vi "SendToSMGRHB.vi"(6 "error in":errorcluster, 7 "meas_point":i32=7, 10 "URL":string="http://smgr.alwaysdata.net/heartbeat/", 11 "date":string="2011-03-24 19:37:00") -> (0 "error out":errorcluster, 2 "body":string="ok", 3 "headers":string="HTTP/1.1 100 Continue\r\n\r\nHTTP/1.1 200 OK\r\nDate: Thu, 24 Mar 2011 13:37:49 GMT\r\nServer: Apache/2.2\r\nVary: Accept-Language,Cookie,User-Agent,Accept-Encoding\r\nContent-Language: en-us\r\nTransfer-Encoding: chunked\r\nContent-Type: text/html; charset=utf-8\r\n\r\n")   [LabVIEW 2010]
uses:
  <vilib>/httpClient/MultipartData.ctl
  <vilib>/httpClient/LabVIEWHTTPClient.lvlib
panel:
  in  "Tab Control":enum32{"Page 1", "Page 2"}(tab)
  out "Array":T1[](array[typedef])=[{"Name"="meas_point", "Value"="7", "File"=path "", "Filename"="", "MIME type"="application/octet-stream"}, {"Name"="date", "Value"="2011-03-24 19:37:00", "File"=path "", "Filename"="", "MIME type"="application/octet-stream"}] caption="Данные для формы"
  # "Измеритель сообщает серверу \nо готовности\n----------------------------------------\nЕсли в ответе, в хедерсе есть \nстрока \"HTTP/1.1 200 OK\"\nзначит всё действительно\nсделано правильно"
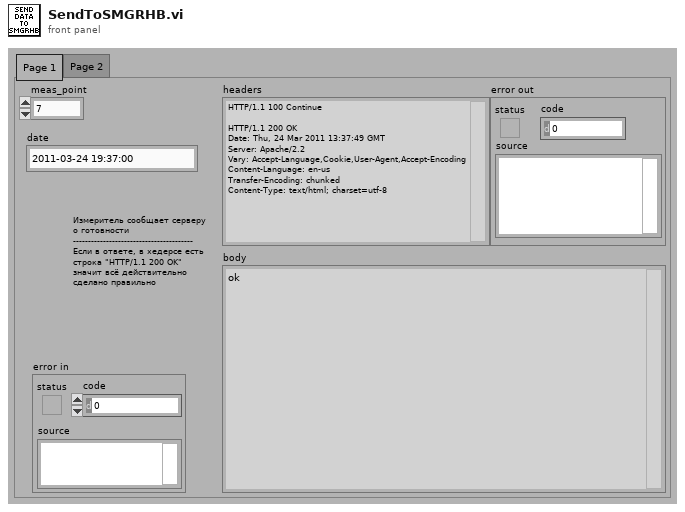
[diagram p1: front panel]
types:
  T1 = typedef "LabVIEWHTTPClient.lvlib/MultipartData.ctl" = cluster{"Name":string, "Value":string, "File":path, "Filename":string, "MIME type":string}
  T2 = typedef "LabVIEWHTTPClient.lvlib/ClientHandle.ctl" = refnum<k1>
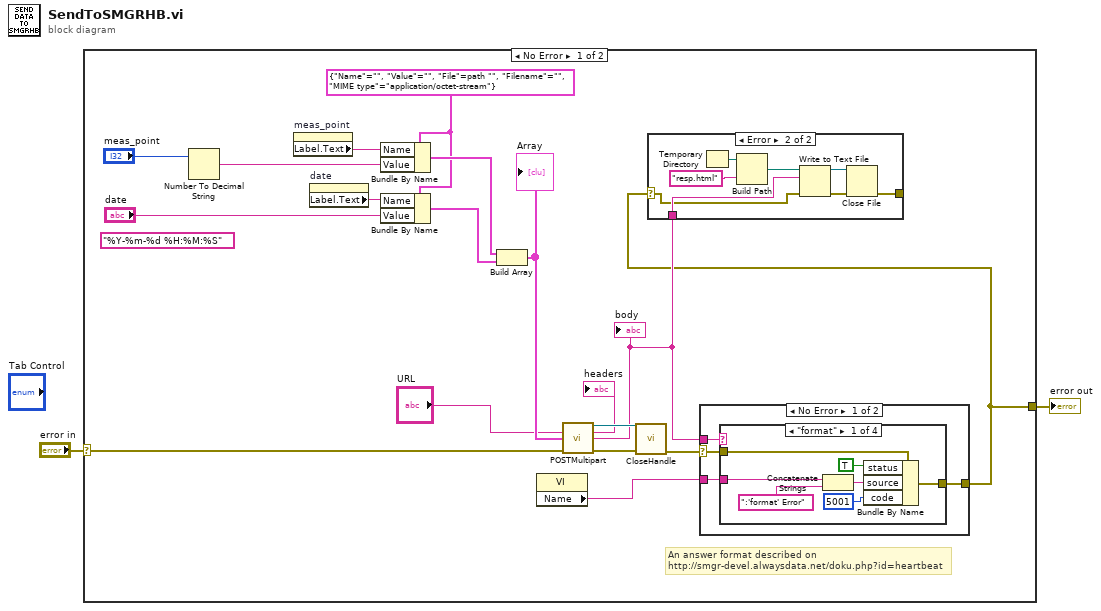
[diagram p0: block diagram]
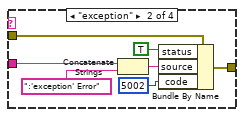
[diagram p2: hidden frame]
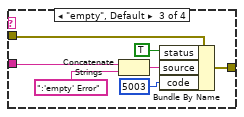
[diagram p3: hidden frame]
diagram:
  n1 = case shown="No Error" "error in" {
    selector: "error in" -> [w13 w57]
    tunnel: [w3 w57] -> w1
    frame No Error {
      w9 = T1 {"Name"="", "Value"="", "File"=path "", "Filename"="", "MIME type"="application/octet-stream"} ("postData")
      (unwired) "%Y-%m-%d %H:%M:%S" ("time format string (%c)")
      # "An answer format described on\nhttp://smgr-devel.alwaysdata.net/doku.php?id=heartbeat"
      n2 = Number To Decimal String(number="meas_point") -> (decimal integer string=w18:string)  [unwired: 1 in]
      n3 = property on="meas_point" class="DigNum (strict)"() -> ("Label.Text"=w15:string)  [unwired: 2 in, 2 out]
      n4 = property on="date" class="Str"() -> ("Label.Text"=w14:string)  [unwired: 2 in, 2 out]
      n5 = Bundle By Name(cluster=w9, "Name"=w15, "Value"=w18) -> (w20:T1)
      n6 = Bundle By Name(cluster=w9, "Name"=w14, "Value"="date") -> (w19:T1)
      n7 = Build Array(w20, w19) -> (w8:T1[])
      "Array" <- w8
      n8 = property on="Property Node" class="VI"() -> ("Name"=w4:string)  [unwired: 2 in, 2 out]
      n9 = call <vilib>:"POSTMultipart.vi"("URL"="URL", "data"=w8, "error in (no error)"=w13) -> ("client handle out"=w12:T2, "headers"=→"headers":string, "body"=w5:string, "error out"=w10:errorcluster)  [unwired: 9 in]
      "body" <- w5
      n10 = call <vilib>:"CloseHandle.vi"("client handle"=w12, "error in (no error)"=w10) -> ("error out"=w6:errorcluster)  [unwired: 13 in]
      n11 = case shown="No Error" w6 {
        selector: w6 -> [w23 w47]
        tunnel: [w22 w47] -> w3
        tunnel: w5 -> [w24 _]
        tunnel: w4 -> [w21 _]
        frame No Error {
          n12 = case shown="\"format\"" w24 {
            tunnel: w23 -> [w29 w33 w41 w46]
            tunnel: [w30 w32 w39 w46] -> w22
            tunnel: w21 -> [w31 w34 w40 _]
            frame "format" {
              n13 = Concatenate Strings(w31, ":'format' Error") -> (w26:string)
              n14 = Bundle By Name(cluster=w29, "status"=TRUE, "source"=w26, "code"=5001) -> (w30:errorcluster)
            }
            frame "exception" {
              n15 = Concatenate Strings(w34, ":'exception' Error") -> (w37:string)
              n16 = Bundle By Name(cluster=w33, "status"=TRUE, "source"=w37, "code"=5002) -> (w32:errorcluster)
            }
            frame "empty", Default {
              n17 = Concatenate Strings(w40, ":'empty' Error") -> (w44:string)
              n18 = Bundle By Name(cluster=w41, "status"=TRUE, "source"=w44, "code"=5003) -> (w39:errorcluster)
            }
            frame "ok" {
            }
          }
        }
        frame Error {
        }
      }
      n19 = case shown="Error" w3 {
        selector: w3 -> [w48 w49]
        tunnel: w5 -> [_ w51]
        tunnel: [w48 w50] -> _
        frame No Error {
        }
        frame Error {
          n20 = Temporary Directory() -> (w56:path)
          n21 = Build Path(base path=w56, name or relative path="resp.html") -> (appended path=w54:path)
          n22 = Write to Text File(file (use dialog)=w54, text=w51, error in=w49) -> (refnum out=w52:refnum<file>, error out=w53:errorcluster)  [unwired: 1 in, 1 out]
          n23 = Close File(refnum=w52, error in=w53) -> (error out=w50:errorcluster)  [unwired: 1 out]
        }
      }
    }
    frame Error {
    }
  }
  "error out" <- w1
